vi "StrainTest.vi"() -> ()   [LabVIEW 2020]
uses:
  <instrlib>/NH Research Regenerative Test Series/Public/Configure/Output Safety.ctl
  Readings.vi
  <instrlib>/NH Research Regenerative Test Series/Public/Data/Read (Ave Current).vi
  <instrlib>/NH Research Regenerative Test Series/Public/Data/Low Level/Fetch (Ave Voltage).vi
  <instrlib>/NH Research Regenerative Test Series/Public/Data/Low Level/Fetch (Ave True Power).vi
  <instrlib>/NH Research Regenerative Test Series/Public/Data/Read (Ave Voltage).vi
  <instrlib>/NH Research Regenerative Test Series/NH Research Regenerative Test Series.lvlib
panel:
  out "Charge Strain":dbl(graph)
  out "Discharge Strain":dbl(graph)
  in  "DWaitStop":bool
  out "Discharge Rest":bool
  in  "Wait Time":u32
  out "Elaspsed Time":u32 caption="Elapsed Time (s)"
  in  "CWait Stop":bool
  out "Charge Rest":bool
  in  "Wait Time":u32
  out "Elapsed Time":u32 caption="Elapsed Time (s)"
  out "Discharge Rest Voltage":dbl
  out "Charge Rest Voltage":dbl
  in  "1C Preset 2":bool
  out "Discharging":bool
  in  "Discharge Stop":bool
  in  "Discharge Current":dbl
  in  "Voltage Cutoff":dbl
  in  "1C Preset":bool
  out "Strain":dbl
  out "Ave Current (A)":dbl
  out "Ave Voltage (V)":dbl
  out "Ave True Power (W)":dbl
  out "Battemp":dbl
  out "AmbientTemp":dbl
  out "Discharge Rest Voltage":dbl(graph)
  out "Charge Rest Voltage":dbl(graph)
  in  "Tab Control":T1(tab)
  out "Selected Output Safety":T2
  in  "Custom Output Safety":T2
  in  "Output Safety\nSelection":bool caption="Output Safety"
  in  "Non Default Folder Path":path
  in  "Cell Number":string
  in  "DAQmx Task Name":refnum<k21>
  in  "NHR VISA Name":refnum<visa-resource-name>
  out "Error Out":string
  out "Previous Discharge Data File":path caption="Filename Out"
  out "File Name":path caption="Filename Out"
  out "D Wait Status Byte Register":T3
  out "Discharge Status Byte Register":T3
  out "C Wait Status Byte Register":T3
  out "Charge Status Byte Register":T3
  out "Task error out":errorcluster
  in  "Cycle Stop":bool
  out "Cycle Index":i32
  in  "Number of Cycles":i32
  out "Charging":bool
  in  "Charge Stop":bool
  in  "Current Cutoff":dbl
  in  "Charge Current":dbl format="%#.6g"
  in  "Charge Voltage":dbl format="%#.6g"
  out "Tab Control 2":T1(tab)
  in  "Logical Instrument Number":u32=1
  # "Readings"
  # "Cycle & Charge Profile Settings"
  # "Charging"
  # "Discharging"
  # "Post Charge\nRest"
  # "Post Discharge\nRest"
  # "Cycle\nInfo"
  # "Rest Voltage Charts"
  # "Output Safety Configuration"
  # "Test Name & Device Info"
  # "Error Indication"
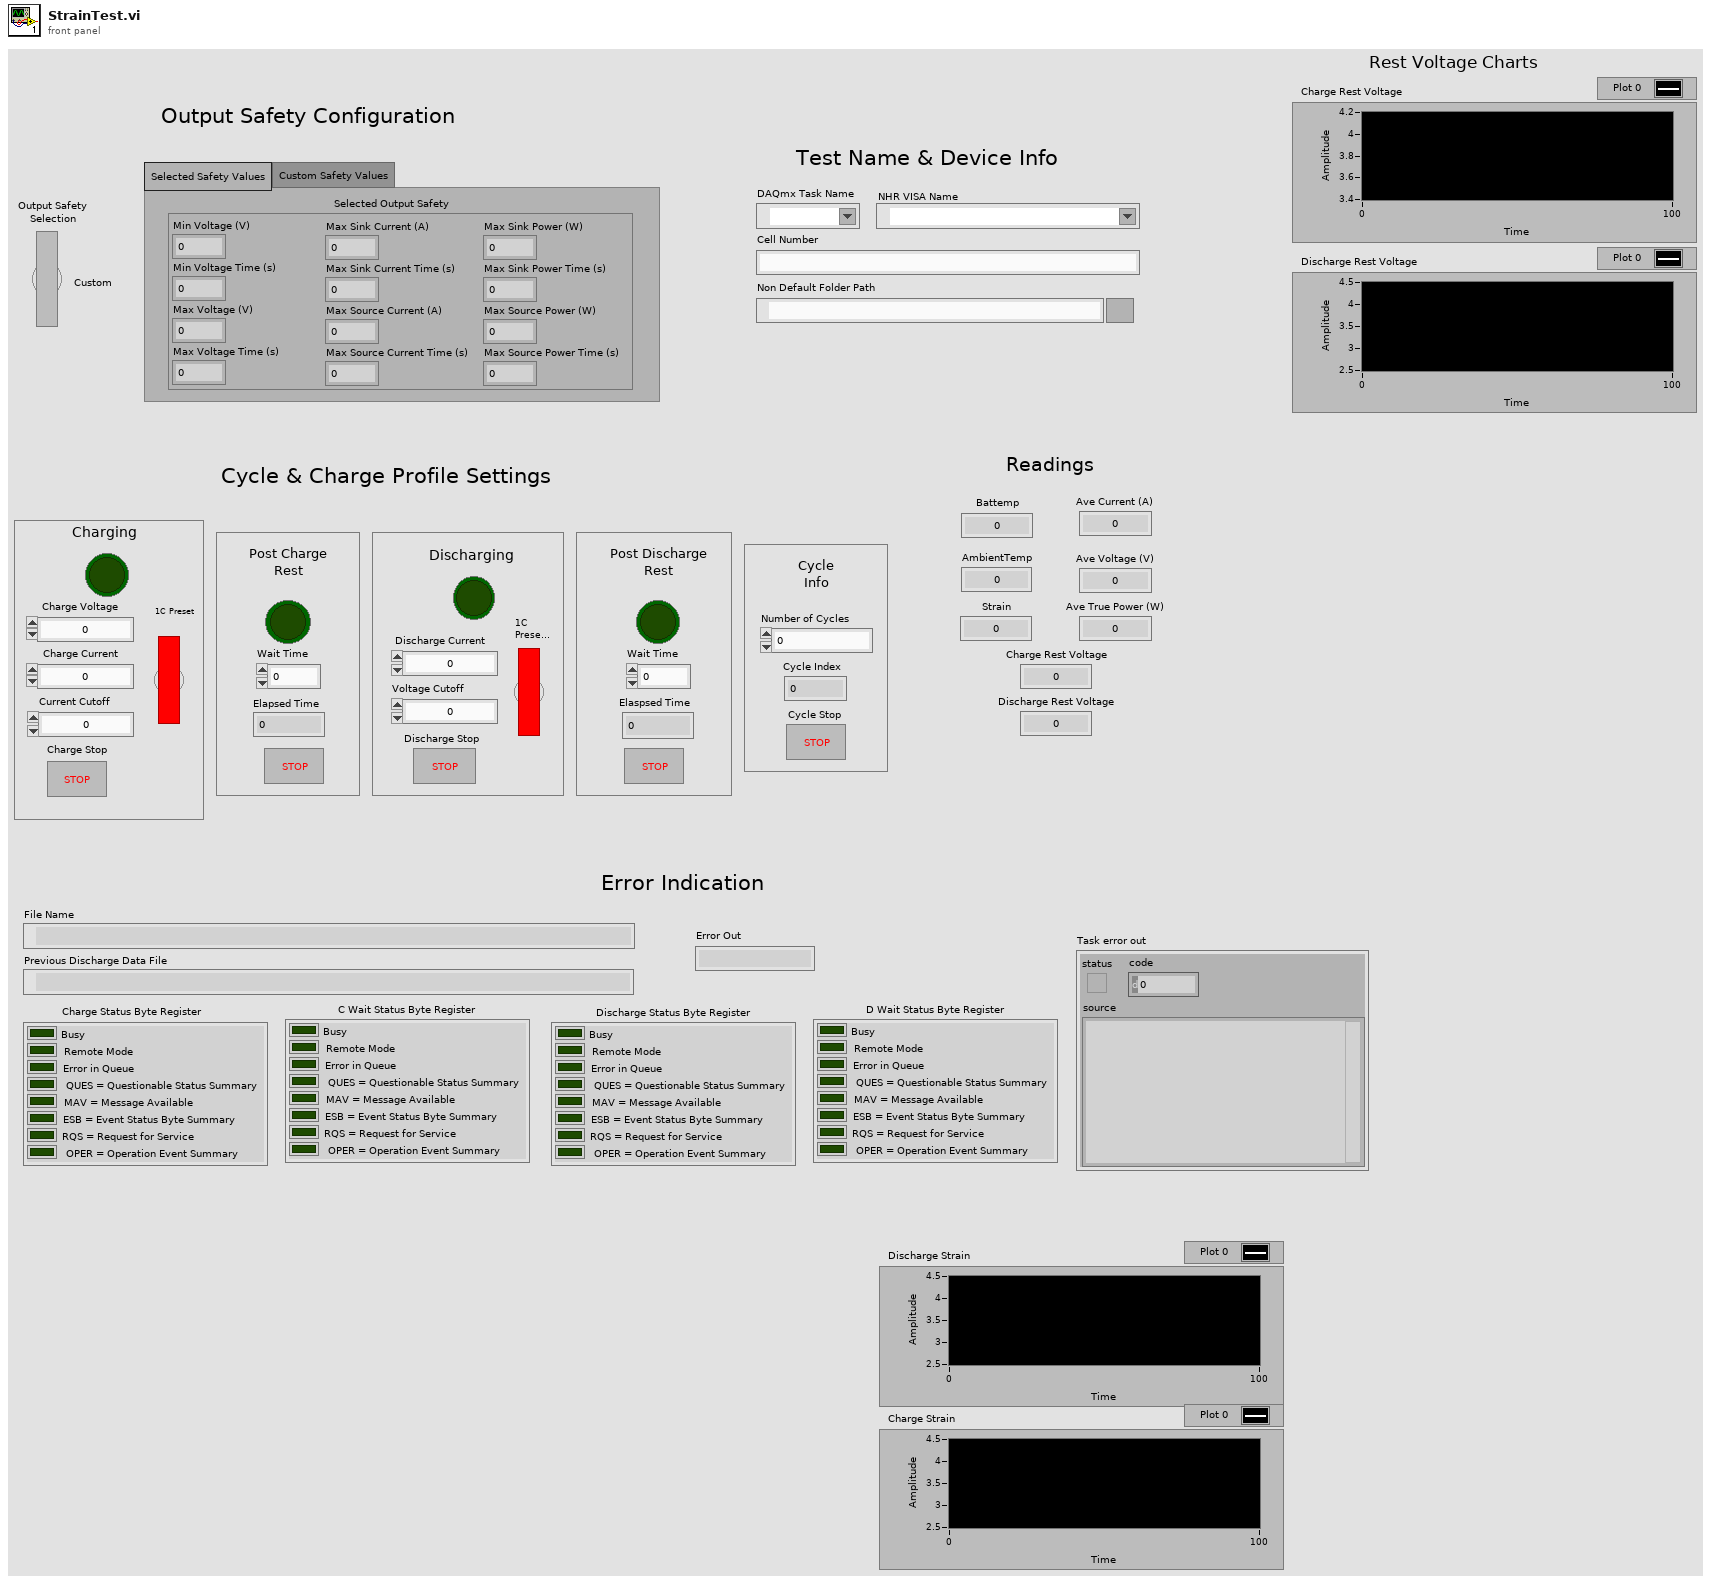
[diagram p1: front panel]
types:
  T1 = enum32{"Selected Safety Values", "Custom Safety Values"}
  T2 = typedef "NH Research Regenerative Test Series.lvlib/Output Safety.ctl" = cluster{"Min Voltage (V)":dbl, "Min Voltage Time (s)":dbl, "Max Voltage (V)":dbl, "Max Voltage Time (s)":dbl, "Max Sink Current (A)":dbl, "Max Sink Current Time (s)":dbl, "Max Source Current (A)":dbl, "Max Source Current Time (s)":dbl, "Max Sink Power (W)":dbl, "Max Sink Power Time (s)":dbl, "Max Source Power (W)":dbl, "Max Source Power Time (s)":dbl}
  T3 = cluster{"Busy":bool, "Remote Mode":bool, "Error in Queue":bool, "QUES = Questionable Status Summary":bool, "MAV = Message Available":bool, "ESB = Event Status Byte Summary":bool, "RQS = Request for Service":bool, "OPER = Operation Event Summary":bool}
  T4 = cluster{"Min Voltage (V)":dbl, "Min Voltage Time (s)":dbl, "Max Voltage (V)":dbl, "Max Voltage Time (s)":dbl, "Max Sink Current (A)":dbl, "Max Sink Current Time (s)":dbl, "Max Source Current (A)":dbl, "Max Source Current Time (s)":dbl, "Max Sink Power (W)":dbl, "Max Sink Power Time (s)":dbl, "Max Source Power (W)":dbl, "Max Source Power Time (s)":dbl}
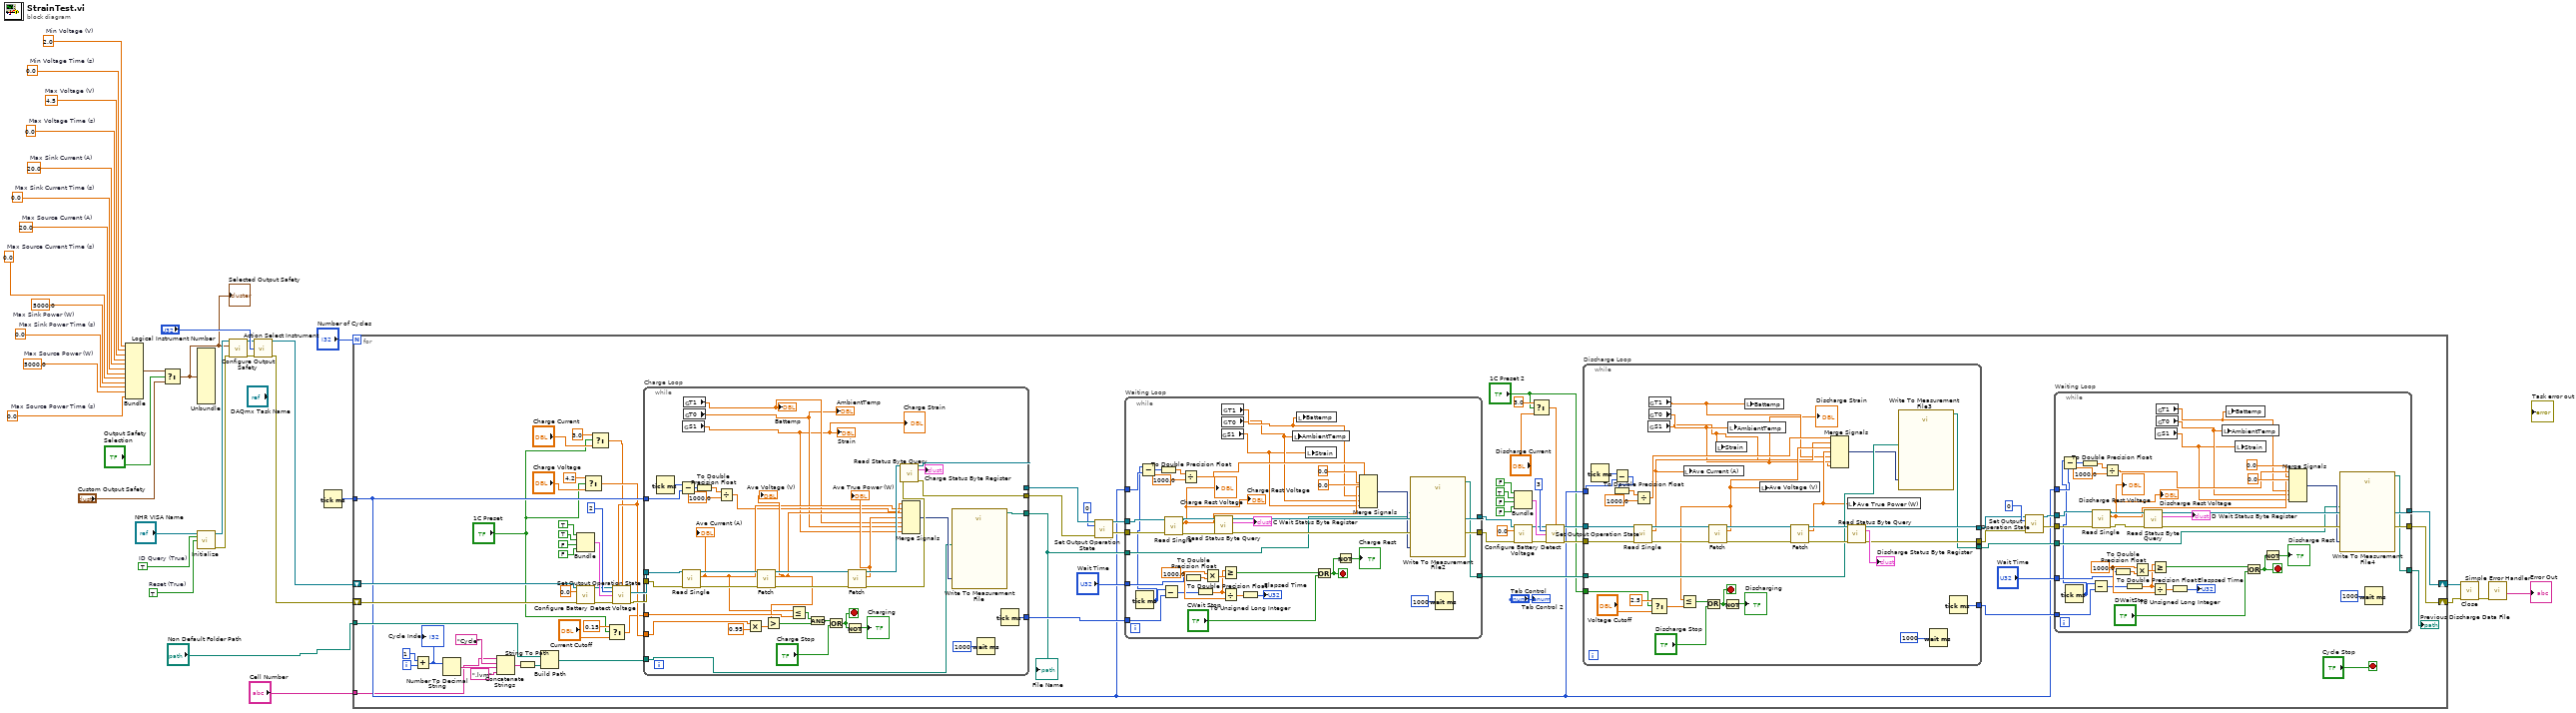
[diagram p0: block diagram]
diagram:
  w9 = 5000.0  # Max Source Power (W)
  w10 = 0.0  # Max Sink Power Time (s)
  w11 = 5000.0  # Max Sink Power (W)
  w12 = 0.0  # Max Source Current Time (s)
  w13 = 20.0  # Max Source Current (A)
  w15 = 20.0  # Max Sink Current (A)
  w14 = 0.0  # Max Sink Current Time (s)
  w16 = 0.0  # Max Voltage Time (s)
  w17 = 4.5  # Max Voltage (V)
  w18 = 2.0  # Min Voltage (V)
  w8 = 0.0  # Max Source Power Time (s)
  w19 = 0.0  # Min Voltage Time (s)
  w33 = TRUE  # ID Query (True)
  w32 = TRUE  # Reset (True)
  n1 = Bundle("Min Voltage (V)"=w18, "Min Voltage Time (s)"=w19, "Max Voltage (V)"=w17, "Max Voltage Time (s)"=w16, "Max Sink Current (A)"=w15, "Max Sink Current Time (s)"=w14, "Max Source Current (A)"=w13, "Max Source Current Time (s)"=w12, "Max Sink Power (W)"=w11, "Max Sink Power Time (s)"=w10, "Max Source Power (W)"=w9, "Max Source Power Time (s)"=w8) -> (w6:T4)  [unwired: 1 in]
  n2 = Select(t=w6, s="Output Safety\nSelection", f="Custom Output Safety") -> (s? t:f=w7:T2)
  "Selected Output Safety" <- w7
  n3 = Unbundle(w7) -> ()  [unwired: 12 out]
  n4 = call <vilib>:"Initialize.vi"("VISA resource name"="NHR VISA Name", "ID Query (True)"=w33, "Reset (True)"=w32) -> ("VISA resource name out"=w31:refnum<visa-resource-name>, "error out"=w30:errorcluster)  [unwired: 11 in]
  n5 = call <vilib>:"Configure Output Safety.vi"("VISA resource name"=w31, "Output Safety"=w7, "error in (no error)"=w30) -> ("VISA resource name out"=w28:refnum<visa-resource-name>, "error out"=w27:errorcluster)  [unwired: 11 in]
  n6 = call <instrlib>:"Action Select Instrument.vi"("VISA resource name"=w28, "Logical Instrument Number"="Logical Instrument Number", "error in (no error)"=w27) -> ("VISA resource name out"=w24:refnum<visa-resource-name>, "error out"=w23:errorcluster)  [unwired: 11 in]
  n7 = Tick Count (ms)() -> (millisecond timer value=w3:u32)
  n8 = for {
    N: "Number of Cycles" -> [_]
    shift-right: [w54] -> w22
    shift-left: w24 -> [w84]
    shift-right: [w53] -> w21
    shift-left: w23 -> [w82]
    tunnel: "Non Default Folder Path" -> [w51]
    tunnel: w3 -> [w50]
    tunnel: "Cell Number" -> [w35]
    i -> [w79]
    stop <- "Cycle Stop" stop-if-true
    n9 = Add(x=1, y=w79) -> (x+y=w73:i32)
    "Cycle Index" <- w73
    n10 = Number To Decimal String(number=w73) -> (decimal integer string=w68:string)  [unwired: 1 in]
    n11 = Concatenate Strings(w35, "Cycle", w68, ".lvm") -> (w74:string)
    n12 = String To Path(string=w74) -> (path=w75:path)
    n13 = Build Path(base path=w51, name or relative path=w75) -> (appended path=w70:path)
    n14 = Bundle(TRUE, TRUE, FALSE, FALSE) -> (w85:cluster{bool, bool, bool, bool})  [unwired: 1 in]
    n15 = call <vilib>:"Configure Battery Detect Voltage.vi"("VISA resource name"=w84, "Battery Detect Voltage (0V)"=0.0, "error in (no error)"=w82) -> ("VISA resource name out"=w83:refnum<visa-resource-name>, "error out"=w81:errorcluster)  [unwired: 11 in]
    n16 = Select(t=4.2, s="1C Preset", f="Charge Voltage") -> (s? t:f=w47:dbl)
    n17 = Select(t=3.0, s="1C Preset", f="Charge Current") -> (s? t:f=w46:dbl)
    n18 = Select(t=0.15, s="1C Preset", f="Current Cutoff") -> (s? t:f=w42:dbl)
    n19 = call <vilib>:"Set Output Operation State.vi"("VISA resource name"=w83, "Voltage Setpoint (0 V)"=w47, "Current Setpoint (0 A)"=w46, "Mode (0: Off)"=2, "Enable"=w85, "error in (no error)"=w81) -> ("VISA resource name out"=w91:refnum<visa-resource-name>, "error out"=w90:errorcluster)  [unwired: 8 in]
    n20 = while "Charge Loop" {
      tunnel: w91 -> [w248]
      tunnel: w90 -> [w247]
      tunnel: [w245] -> w96
      tunnel: [w244] -> w95
      tunnel: w42 -> [w240]
      tunnel: w70 -> [w235]
      tunnel: [w241] -> w64
      tunnel: [w236] -> w78
      tunnel: w47 -> [w227]
      tunnel: w50 -> [w225]
      stop <- w232 stop-if-true
      n21 = Tick Count (ms)() -> (millisecond timer value=w226:u32)
      n22 = Subtract(x=w226, y=w225) -> (x-y=w224:u32)
      n23 = call-poly <instrlib>:"Read Single.vi"("VISA resource name"=w248, "error in (no error)"=w247) -> ("VISA resource name out"=w253:refnum<visa-resource-name>, "Ave Current (A)"=w221:dbl, "error out"=w254:errorcluster)  [unwired: 11 in]
      "Ave Current (A)" <- w221
      n24 = global read "Readings.vi" "S1"() -> (w217:dbl)
      "Strain" <- w217
      "Charge Strain" <- w217
      n25 = global read "Readings.vi" "T1"() -> (w219:dbl)
      "Battemp" <- w219
      n26 = global read "Readings.vi" "T0"() -> (w218:dbl)
      "AmbientTemp" <- w218
      n27 = To Double Precision Float(number=w224) -> (double precision float=w222:dbl)
      n28 = Divide(x=w222, y=1000.0) -> (x/y=w220:dbl)
      n29 = Multiply(x=w227, y=0.95) -> (x*y=w229:dbl)
      n30 = call-poly <instrlib>:"Fetch.vi"("VISA resource name"=w253, "error in (no error)"=w254) -> ("VISA resource name out"=w252:refnum<visa-resource-name>, "Ave Voltage (V)"=w230:dbl, "error out"=w251:errorcluster)  [unwired: 11 in]
      "Ave Voltage (V)" <- w230
      n31 = Greater?(x=w230, y=w229) -> (0:w237:bool)
      n32 = Less Or Equal?(x=w221, y=w240) -> (x <= y?=w238:bool)
      n33 = And(x=w238, y=w237) -> (x .and. y?=w234:bool)
      n34 = Or(x=w234, y="Charge Stop") -> (x .or. y?=w232:bool)
      n35 = Not(x=w232) -> (.not. x?=→"Charging":bool)
      n36 = call-poly <instrlib>:"Fetch.vi"("VISA resource name"=w252, "error in (no error)"=w251) -> ("VISA resource name out"=w250:refnum<visa-resource-name>, "Ave True Power (W)"=w243:dbl, "error out"=w249:errorcluster)  [unwired: 11 in]
      "Ave True Power (W)" <- w243
      n37 = call <instrlib>:"Read Status Byte Query.vi"("VISA resource name"=w250, "error in (no error)"=w249) -> ("VISA resource name out"=w245:refnum<visa-resource-name>, "Status Byte Register"=→"Charge Status Byte Register":T3, "error out"=w244:errorcluster)  [unwired: 11 in]
      n38 = Merge Signals "Merge Signals"(w220, w221, w230, w243, w219, w218, w217) -> (w242:dynamicdata)
      n39 = call "Write To Measurement File"("Signals"=w242, "Filename"=w235) -> ("Filename Out"=w241:path)  [unwired: 15 in, 2 out]
      n40 = Wait (ms)(milliseconds to wait=u32 1000) -> ()  [unwired: 1 out]
      n41 = Tick Count (ms)() -> (millisecond timer value=w236:u32)
    }
    "File Name" <- w64
    n42 = call <vilib>:"Set Output Operation State.vi"("VISA resource name"=w96, "Mode (0: Off)"=0, "error in (no error)"=w95) -> ("VISA resource name out"=w93:refnum<visa-resource-name>, "error out"=w66:errorcluster)  [unwired: 11 in]
    n43 = while "Waiting Loop" {
      tunnel: [w215] -> w98
      tunnel: "Wait Time" -> [w205]
      tunnel: w78 -> [w212]
      tunnel: w93 -> [w195]
      tunnel: w66 -> [w194]
      tunnel: [w203] -> w65
      tunnel: w64 -> [w200]
      tunnel: [w199] -> w63
      tunnel: w50 -> [w193]
      stop <- w184 stop-if-true
      w213 = 1000.0
      n44 = Tick Count (ms)() -> (millisecond timer value=w192:u32)
      n45 = Subtract(x=w192, y=w193) -> (x-y=w189:u32)
      n46 = To Double Precision Float(number=w189) -> (double precision float=w190:dbl)
      n47 = Subtract(x=w192, y=w212) -> (x-y=w207:u32)
      n48 = call-poly <instrlib>:"Read Single.vi"("VISA resource name"=w195, "error in (no error)"=w194) -> ("VISA resource name out"=w197:refnum<visa-resource-name>, "Ave Voltage (V)"=w196:dbl, "error out"=w198:errorcluster)  [unwired: 11 in]
      "Charge Rest Voltage" <- w196
      "Charge Rest Voltage" <- w196
      n49 = Divide(x=w190, y=1000.0) -> (x/y=w187:dbl)
      n50 = To Double Precision Float(number=w205) -> (double precision float=w204:dbl)
      n51 = To Double Precision Float(number=w207) -> (double precision float=w206:dbl)
      n52 = Multiply(x=w213, y=w204) -> (x*y=w214:dbl)
      n53 = call <instrlib>:"Read Status Byte Query.vi"("VISA resource name"=w197, "error in (no error)"=w198) -> ("VISA resource name out"=w215:refnum<visa-resource-name>, "Status Byte Register"=→"C Wait Status Byte Register":T3, "error out"=w203:errorcluster)  [unwired: 11 in]
      n54 = global read "Readings.vi" "S1"() -> (w181:dbl)
      n55 = global read "Readings.vi" "T1"() -> (w183:dbl)
      n56 = global read "Readings.vi" "T0"() -> (w182:dbl)
      n57 = Greater Or Equal?(x=w206, y=w214) -> (x >= y?=w186:bool)
      n58 = Divide(x=w206, y=w213) -> (x/y=w209:dbl)
      n59 = To Unsigned Long Integer(number=w209) -> (unsigned 32bit integer=→"Elapsed Time":u32)
      n60 = local write "AmbientTemp"(w182) -> ()
      n61 = local write "Battemp"(w183) -> ()
      n62 = local write "Strain"(w181) -> ()
      n63 = Or(x=w186, y="CWait Stop") -> (x .or. y?=w184:bool)
      n64 = Not(x=w184) -> (.not. x?=→"Charge Rest":bool)
      n65 = Merge Signals "Merge Signals"(w187, 0.0, w196, 0.0, w183, w182, w181) -> (w201:dynamicdata)
      n66 = call "Write To Measurement File2"("Signals"=w201, "Filename"=w200) -> ("Filename Out"=w199:path)  [unwired: 15 in, 2 out]
      n67 = Wait (ms)(milliseconds to wait=u32 1000) -> ()  [unwired: 1 out]
    }
    n68 = Bundle(FALSE, TRUE, FALSE, FALSE) -> (w100:cluster{bool, bool, bool, bool})  [unwired: 1 in]
    n69 = call <vilib>:"Configure Battery Detect Voltage.vi"("VISA resource name"=w98, "Battery Detect Voltage (0V)"=0.0, "error in (no error)"=w65) -> ("VISA resource name out"=w97:refnum<visa-resource-name>, "error out"=w99:errorcluster)  [unwired: 11 in]
    n70 = Select(t=3.0, s="1C Preset 2", f="Discharge Current") -> (s? t:f=w37:dbl)
    n71 = call <vilib>:"Set Output Operation State.vi"("VISA resource name"=w97, "Current Setpoint (0 A)"=w37, "Mode (0: Off)"=3, "Enable"=w100, "error in (no error)"=w99) -> ("VISA resource name out"=w105:refnum<visa-resource-name>, "error out"=w106:errorcluster)  [unwired: 9 in]
    n72 = while "Discharge Loop" {
      tunnel: w105 -> [w174]
      tunnel: w106 -> [w173]
      tunnel: [w171] -> w58
      tunnel: [w170] -> w59
      tunnel: w63 -> [w169]
      tunnel: [w157] -> w57
      tunnel: [w160] -> w56
      tunnel: w50 -> [w158]
      tunnel: "1C Preset 2" -> [w148]
      stop <- w163 stop-if-true
      n73 = Tick Count (ms)() -> (millisecond timer value=w159:u32)
      n74 = Subtract(x=w159, y=w158) -> (x-y=w154:u32)
      n75 = To Double Precision Float(number=w154) -> (double precision float=w155:dbl)
      n76 = call-poly <instrlib>:"Read Single.vi"("VISA resource name"=w174, "error in (no error)"=w173) -> ("VISA resource name out"=w179:refnum<visa-resource-name>, "Ave Current (A)"=w153:dbl, "error out"=w180:errorcluster)  [unwired: 11 in]
      n77 = Divide(x=w155, y=1000.0) -> (x/y=w152:dbl)
      n78 = global read "Readings.vi" "S1"() -> (w145:dbl)
      "Discharge Strain" <- w145
      n79 = global read "Readings.vi" "T1"() -> (w147:dbl)
      n80 = global read "Readings.vi" "T0"() -> (w146:dbl)
      n81 = Select(t=2.5, s=w148, f="Voltage Cutoff") -> (s? t:f=w149:dbl)
      n82 = local write "Ave Current (A)"(w153) -> ()
      n83 = call-poly <instrlib>:"Fetch.vi"("VISA resource name"=w179, "error in (no error)"=w180) -> ("VISA resource name out"=w178:refnum<visa-resource-name>, "Ave Voltage (V)"=w162:dbl, "error out"=w177:errorcluster)  [unwired: 11 in]
      n84 = Less Or Equal?(x=w162, y=w149) -> (x <= y?=w166:bool)
      n85 = Or(x=w166, y="Discharge Stop") -> (x .or. y?=w163:bool)
      n86 = local write "Strain"(w145) -> ()
      n87 = Not(x=w163) -> (.not. x?=→"Discharging":bool)
      n88 = local write "AmbientTemp"(w146) -> ()
      n89 = local write "Battemp"(w147) -> ()
      n90 = local write "Ave Voltage (V)"(w162) -> ()
      n91 = call-poly <instrlib>:"Fetch.vi"("VISA resource name"=w178, "error in (no error)"=w177) -> ("VISA resource name out"=w176:refnum<visa-resource-name>, "Ave True Power (W)"=w161:dbl, "error out"=w175:errorcluster)  [unwired: 11 in]
      n92 = Merge Signals "Merge Signals"(w152, w153, w162, w161, w147, w146, w145) -> (w168:dynamicdata)
      n93 = local write "Ave True Power (W)"(w161) -> ()
      n94 = call <instrlib>:"Read Status Byte Query.vi"("VISA resource name"=w176, "error in (no error)"=w175) -> ("VISA resource name out"=w171:refnum<visa-resource-name>, "Status Byte Register"=→"Discharge Status Byte Register":T3, "error out"=w170:errorcluster)  [unwired: 11 in]
      n95 = call "Write To Measurement File3"("Signals"=w168, "Filename"=w169) -> ("Filename Out"=w160:path)  [unwired: 15 in, 2 out]
      n96 = Wait (ms)(milliseconds to wait=u32 1000) -> ()  [unwired: 1 out]
      n97 = Tick Count (ms)() -> (millisecond timer value=w157:u32)
    }
    n98 = call <vilib>:"Set Output Operation State.vi"("VISA resource name"=w58, "Mode (0: Off)"=0, "error in (no error)"=w59) -> ("VISA resource name out"=w62:refnum<visa-resource-name>, "error out"=w61:errorcluster)  [unwired: 11 in]
    n99 = while "Waiting Loop" {
      tunnel: [w144] -> w54
      tunnel: "Wait Time" -> [w136]
      tunnel: w57 -> [w141]
      tunnel: w62 -> [w126]
      tunnel: w61 -> [w125]
      tunnel: [w134] -> w53
      tunnel: [w131] -> w52
      tunnel: w56 -> [w130]
      tunnel: w50 -> [w121]
      stop <- w112 stop-if-true
      w142 = 1000.0
      n100 = Tick Count (ms)() -> (millisecond timer value=w120:u32)
      n101 = Subtract(x=w120, y=w121) -> (x-y=w117:u32)
      n102 = To Double Precision Float(number=w117) -> (double precision float=w118:dbl)
      n103 = Subtract(x=w120, y=w141) -> (x-y=w138:u32)
      n104 = call-poly <instrlib>:"Read Single.vi"("VISA resource name"=w126, "error in (no error)"=w125) -> ("VISA resource name out"=w124:refnum<visa-resource-name>, "Ave Voltage (V)"=w123:dbl, "error out"=w122:errorcluster)  [unwired: 11 in]
      "Discharge Rest Voltage" <- w123
      "Discharge Rest Voltage" <- w123
      n105 = Divide(x=w118, y=1000.0) -> (x/y=w116:dbl)
      n106 = To Double Precision Float(number=w136) -> (double precision float=w135:dbl)
      n107 = To Double Precision Float(number=w138) -> (double precision float=w137:dbl)
      n108 = Multiply(x=w142, y=w135) -> (x*y=w143:dbl)
      n109 = call <instrlib>:"Read Status Byte Query.vi"("VISA resource name"=w124, "error in (no error)"=w122) -> ("VISA resource name out"=w144:refnum<visa-resource-name>, "Status Byte Register"=→"D Wait Status Byte Register":T3, "error out"=w134:errorcluster)  [unwired: 11 in]
      n110 = Greater Or Equal?(x=w137, y=w143) -> (x >= y?=w114:bool)
      n111 = Divide(x=w137, y=w142) -> (x/y=w139:dbl)
      n112 = global read "Readings.vi" "S1"() -> (w109:dbl)
      n113 = global read "Readings.vi" "T1"() -> (w111:dbl)
      n114 = global read "Readings.vi" "T0"() -> (w110:dbl)
      n115 = To Unsigned Long Integer(number=w139) -> (unsigned 32bit integer=→"Elaspsed Time":u32)
      n116 = local write "AmbientTemp"(w110) -> ()
      n117 = local write "Battemp"(w111) -> ()
      n118 = local write "Strain"(w109) -> ()
      n119 = Or(x=w114, y="DWaitStop") -> (x .or. y?=w112:bool)
      n120 = Not(x=w112) -> (.not. x?=→"Discharge Rest":bool)
      n121 = Merge Signals "Merge Signals"(w116, 0.0, w123, 0.0, w111, w110, w109) -> (w132:dynamicdata)
      n122 = call "Write To Measurement File4"("Signals"=w132, "Filename"=w130) -> ("Filename Out"=w131:path)  [unwired: 15 in, 2 out]
      n123 = Wait (ms)(milliseconds to wait=u32 1000) -> ()  [unwired: 1 out]
    }
    "Previous Discharge Data File" <- w52
    "Tab Control 2" <- "Tab Control"
  }
  n124 = call <instrlib>:"Close.vi"("VISA resource name"=w22, "error in (no error)"=w21) -> ("error out"=w26:errorcluster)  [unwired: 13 in]
  n125 = call <vilib>:"Simple Error Handler.vi"("error in (no error)"=w26) -> ("source out"=→"Error Out":string)  [unwired: 4 in, 4 out]
